vi "New Terminal.vi"(5 "Terminal in":refnum<class "SMOTerminal.lvclass">, 8 "error in (no error)":errorcluster, 10 "Required":bool, 11 "Control Reference":refnum<vi>) -> (0 "error out":errorcluster, 2 "Supported type":bool, 3 "Terminal out":refnum<class "SMOTerminal.lvclass">)   [LabVIEW 2013, in "SMOTerminal.lvclass"]
uses:
  SMOTerminal.lvclass
  <vilib>/Utility/VariantDataType/Type.ctl
  SMOTerminal.lvclass/SMOTerminal.ctl
  <vilib>/Utility/VariantDataType/VariantType.lvlib
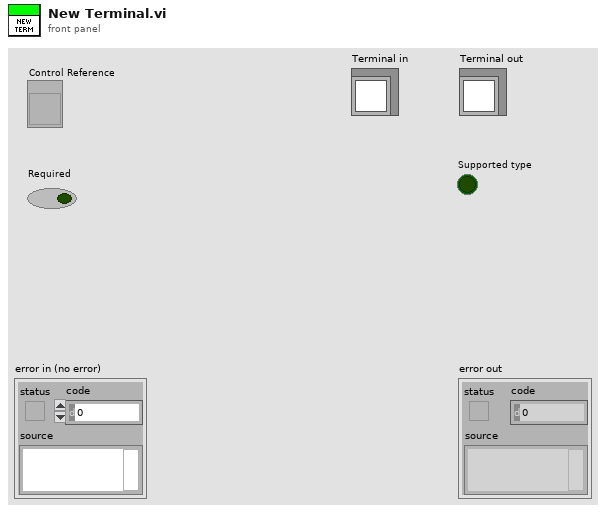
[diagram p1: front panel]
types:
  T1 = typedef "VariantType.lvlib/Type.ctl" = enum8{"Invalid Type", "Void", "I8", "I16", "I32", "I64", "U8", "U16", "U32", "U64", "Single Float", "Double Float", "Extended Float", "Single Complex", "Double Complex", "Extended Complex", "Enum U8", "Enum U16", "Enum U32", "Enum U64", "Single Float With Unit", "Double Float With Unit", "Extended Float With Unit", "Single Complex with Unit", "Double Complex with Unit", "Extended Complex with Unit", "Boolean", "String", "Path", "Picture", "Tag", "Array", "Cluster", "Variant", "LV Variant", "Waveform", "Timestamp", "Digital Waveform", "Digital Data", "ExpressData", "Refnum", "External Data", "VI", "Poly VI", "LabVIEW Class Instance", "Fixed Point"}
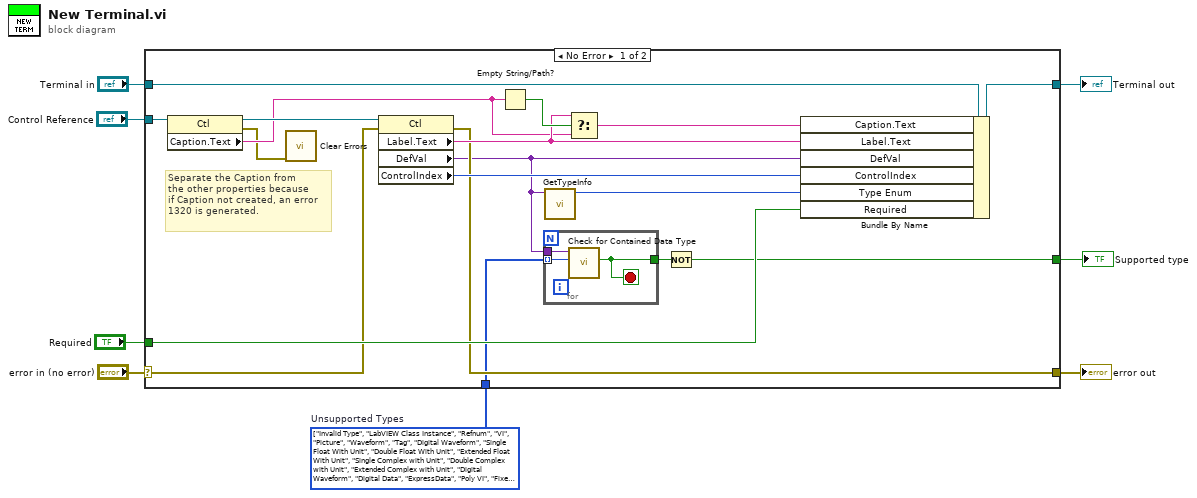
[diagram p0: block diagram]
diagram:
  w2 = T1[] [enum."Invalid Type", enum."LabVIEW Class Instance", enum."Refnum", enum."VI", enum."Picture", enum."Waveform", enum."Tag", enum."Digital Waveform", enum."Single Float With Unit", enum."Double Float With Unit", enum."Extended Float With Unit", enum."Single Complex with Unit", enum."Double Complex with Unit", enum."Extended Complex with Unit", enum."Digital Waveform", enum."Digital Data", enum."ExpressData", enum."Poly VI", enum."Fixed Point"] items=["Invalid Type", "Void", "I8", "I16", "I32", "I64", "U8", "U16", "U32", "U64", "Single Float", "Double Float", "Extended Float", "Single Complex", "Double Complex", "Extended Complex", "Enum U8", "Enum U16", "Enum U32", "Enum U64", "Single Float With Unit", "Double Float With Unit", "Extended Float With Unit", "Single Complex with Unit", "Double Complex with Unit", "Extended Complex with Unit", "Boolean", "String", "Path", "Picture", "Tag", "Array", "Cluster", "Variant", "LV Variant", "Waveform", "Timestamp", "Digital Waveform", "Digital Data", "ExpressData", "Refnum", "External Data", "VI", "Poly VI", "LabVIEW Class Instance", "Fixed Point"]  # Unsupported Types
  n1 = case shown="No Error" "error in (no error)" {
    selector: "error in (no error)" -> [w20 w31]
    tunnel: [w19 w31] -> w7
    tunnel: [w25 w30] -> w5
    tunnel: "Terminal in" -> [w26 w30]
    tunnel: "Control Reference" -> [w18 _]
    tunnel: "Required" -> [w21 _]
    tunnel: w2 -> [w12 _]
    tunnel: [w10 _] -> w1
    frame No Error {
      # "Separate the Caption from\nthe other properties because\nif Caption not created, an error\n1320 is generated."
      n2 = property class="Ctl"(reference=w18) -> (reference out=w17:refnum<vi>, error out=w14:errorcluster, "Caption.Text"=w15:string)  [unwired: 1 in]
      n3 = call <vilib>:"Clear Errors.vi"("error in (no error)"=w14) -> ()  [unwired: 6 in, 1 out]
      n4 = property class="Ctl"(reference=w17, error in=w20) -> (error out=w19:errorcluster, "Label.Text"=w23:string, "DefVal"=w13:variant, "ControlIndex"=w22:i32)  [unwired: 1 out]
      n5 = Empty String/Path?(string/path=w15) -> (empty?=w24:bool)
      n6 = for {
        tunnel: w13 -> [w29]
        tunnel: w12 -> [w28] mode=indexing
        tunnel: [w27] -> w11
        stop <- w27 stop-if-true
        n7 = call <vilib>:"Check for Contained Data Type.vi"("Data Type to Find"=w28, "Data Type"=w29) -> ("Contains Data Type to Find?"=w27:bool)  [unwired: 7 in, 2 out]
      }
      n8 = call <vilib>:"GetTypeInfo.vi"("Variant"=w13) -> ("Type Enum"=w9:T1)  [unwired: 6 in, 4 out]
      n9 = Select(t=w23, s=w24, f=w15) -> (s? t:f=w16:string)
      n10 = Not(x=w11) -> (.not. x?=w10:bool)
      n11 = Bundle By Name(cluster=w26, "Caption.Text"=w16, "Label.Text"=w23, "DefVal"=w13, "ControlIndex"=w22, "Type Enum"=w9, "Required"=w21) -> (w25:refnum<class "SMOTerminal.lvclass">)
    }
    frame Error {
    }
  }
  "error out" <- w7
  "Terminal out" <- w5
  "Supported type" <- w1
